vi "Project.vi"() -> ()   [LabVIEW 2023]
uses:
  WasherDryerControl.ctl
panel:
  out "Duration in hours":dbl
  out "Window":dbl(knob) scale=0.0..1000.0
  out "Temp":dbl
  out "Count":i32
  out "State":T1=enum."DO IT, ANAKIN"
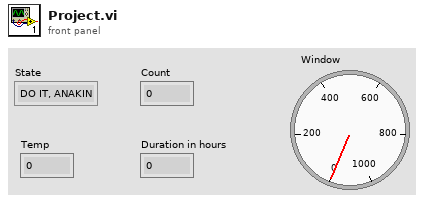
[diagram p1: front panel]
types:
  T1 = typedef "WasherDryerControl.ctl" = enum16{"Start", "Stop", "Wait", "Wash", "Cycle", "400", "800", "1200", "Temp", "Dry", "Heat", "Dry Flat", "Low heat", "High Heat", "Duration", "1h", "2h", "DO IT, ANAKIN"}
  T2 = enum16{"Left Button", "Center Button", "Right Button", "Window Close"}
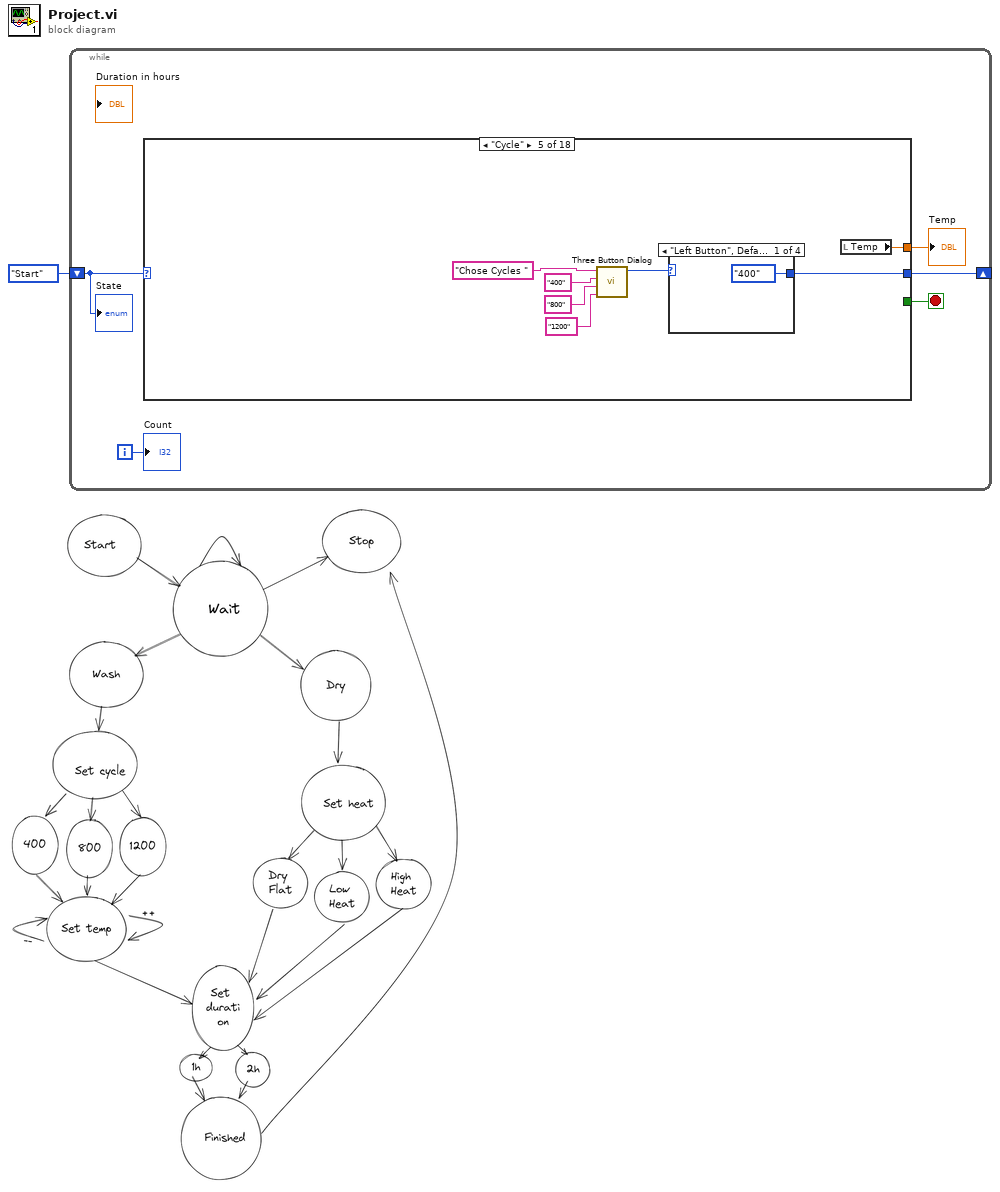
[diagram p0: block diagram]
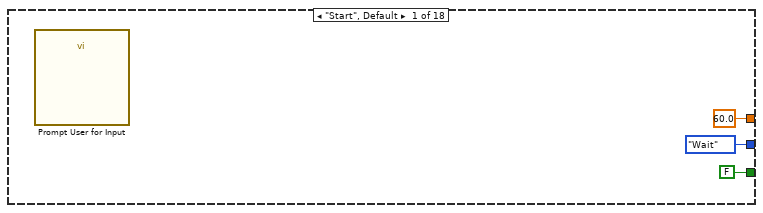
[diagram p2: hidden frame]
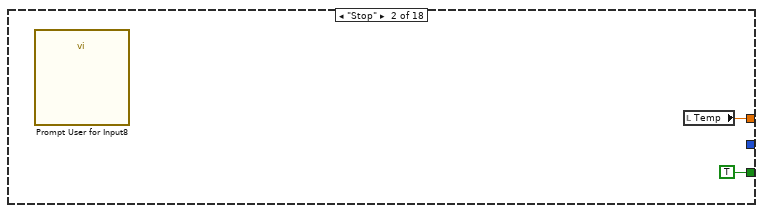
[diagram p3: hidden frame]
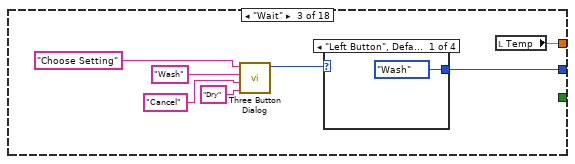
[diagram p4: hidden frame]
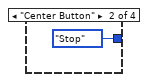
[diagram p5: hidden frame]
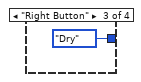
[diagram p6: hidden frame]
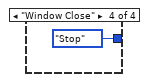
[diagram p7: hidden frame]
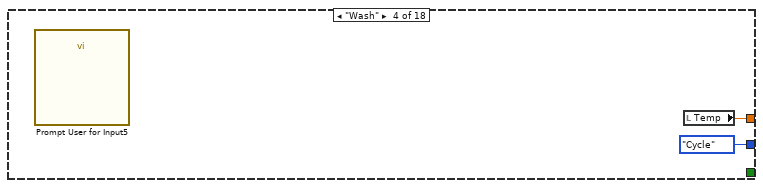
[diagram p8: hidden frame]
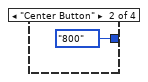
[diagram p9: hidden frame]
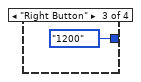
[diagram p10: hidden frame]
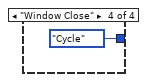
[diagram p11: hidden frame]
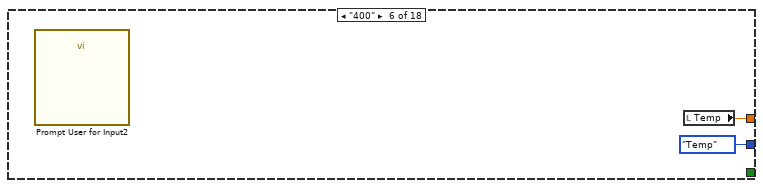
[diagram p12: hidden frame]
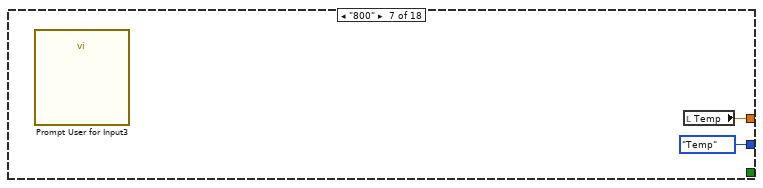
[diagram p13: hidden frame]
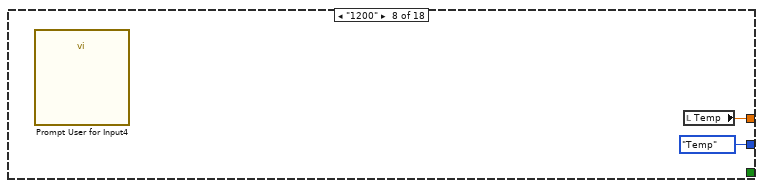
[diagram p14: hidden frame]
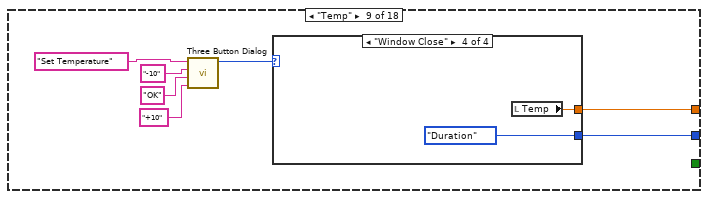
[diagram p15: hidden frame]
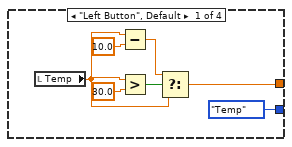
[diagram p16: hidden frame]
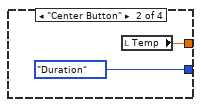
[diagram p17: hidden frame]
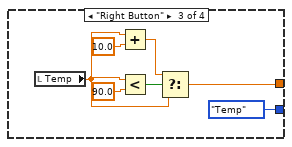
[diagram p18: hidden frame]
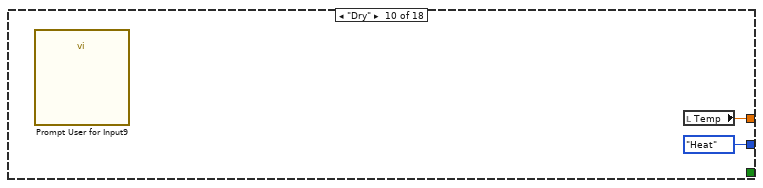
[diagram p19: hidden frame]
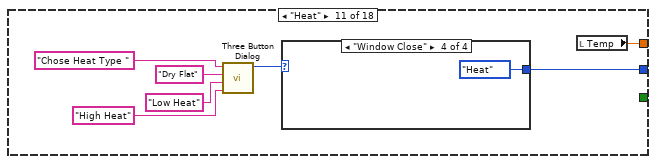
[diagram p20: hidden frame]
diagram:
  n1 = while {
    shift-right: [w3] -> _
    shift-left: WasherDryerControl."Start" ("Enum 2") -> [w4]
    i -> [w6]
    stop <- w5 stop-if-true
    n2 = case shown="\"Cycle\"" w4 {
      tunnel: [FALSE TRUE _ _ _ _ _ _ _ _ _ _ _ _ _ _ _ _] -> w5
      tunnel: [WasherDryerControl."Wait" ("Enum 2") _ w17 WasherDryerControl."Cycle" ("Enum 2") w29 WasherDryerControl."Temp" ("Enum 2") WasherDryerControl."Temp" ("Enum 2") WasherDryerControl."Temp" ("Enum 2") w43 WasherDryerControl."Heat" ("Enum 2") w70 WasherDryerControl."Duration" ("Enum 2") WasherDryerControl."Duration" ("Enum 2") WasherDryerControl."Duration" ("Enum 2") w87 WasherDryerControl."DO IT, ANAKIN" ("Enum 2") WasherDryerControl."DO IT, ANAKIN" ("Enum 2") w101] -> w3
      tunnel: [60.0 ("Temp") w10 w12 w23 w25 w36 w38 w40 w42 w67 w69 0.0 ("Temp") 30.0 ("Temp") 90.0 ("Temp") w86 w94 w97 w100] -> w2
      frame "Start", Default {
        n3 = call "Prompt User for Input"() -> ()  [unwired: 18 in, 2 out]
      }
      frame "Stop" {
        n4 = call "Prompt User for Input8"() -> ()  [unwired: 18 in, 2 out]
        n5 = local read "Temp"() -> (w10:dbl)
      }
      frame "Wait" {
        n6 = call <vilib>:"Three Button Dialog.vi"("Right Button Text (\"Cancel\")"="Dry" ("Right Button Text (\"Cancel\")"), "Center Button Text (\"No\")"="Cancel" ("Center Button Text (\"No\")"), "Left Button Text (\"Yes\")"="Wash" ("Left Button Text (\"Yes\")"), "message"="Choose Setting") -> ("Which Button?"=w18:T2)  [unwired: 7 in]
        n7 = case shown="\"Left Button\", Default" w18 {
          tunnel: [WasherDryerControl."Wash" ("Enum 2") WasherDryerControl."Stop" ("Enum 2") WasherDryerControl."Dry" ("Enum 2") WasherDryerControl."Stop" ("Enum 2")] -> w17
          frame "Left Button", Default {
          }
          frame "Center Button" {
          }
          frame "Right Button" {
          }
          frame "Window Close" {
          }
        }
        n8 = local read "Temp"() -> (w12:dbl)
      }
      frame "Wash" {
        n9 = call "Prompt User for Input5"() -> ()  [unwired: 18 in, 2 out]
        n10 = local read "Temp"() -> (w23:dbl)
      }
      frame "Cycle" {
        n11 = call <vilib>:"Three Button Dialog.vi"("Right Button Text (\"Cancel\")"="1200" ("Right Button Text (\"Cancel\")"), "Center Button Text (\"No\")"="800" ("Center Button Text (\"No\")"), "Left Button Text (\"Yes\")"="400" ("Center Button Text (\"No\")"), "message"="Chose Cycles ") -> ("Which Button?"=w31:T2)  [unwired: 7 in]
        n12 = case shown="\"Left Button\", Default" w31 {
          tunnel: [WasherDryerControl."400" ("Enum 2") WasherDryerControl."800" ("Enum 2") WasherDryerControl."1200" ("Enum 2") WasherDryerControl."Cycle" ("Enum 2")] -> w29
          frame "Left Button", Default {
          }
          frame "Center Button" {
          }
          frame "Right Button" {
          }
          frame "Window Close" {
          }
        }
        n13 = local read "Temp"() -> (w25:dbl)
      }
      frame "400" {
        n14 = call "Prompt User for Input2"() -> ()  [unwired: 18 in, 2 out]
        n15 = local read "Temp"() -> (w36:dbl)
      }
      frame "800" {
        n16 = call "Prompt User for Input3"() -> ()  [unwired: 18 in, 2 out]
        n17 = local read "Temp"() -> (w38:dbl)
      }
      frame "1200" {
        n18 = call "Prompt User for Input4"() -> ()  [unwired: 18 in, 2 out]
        n19 = local read "Temp"() -> (w40:dbl)
      }
      frame "Temp" {
        n20 = call <vilib>:"Three Button Dialog.vi"("Right Button Text (\"Cancel\")"="+10" ("Right Button Text (\"Cancel\")"), "Center Button Text (\"No\")"="OK" ("Center Button Text (\"No\")"), "Left Button Text (\"Yes\")"="-10" ("Left Button Text (\"Yes\")"), "message"="Set Temperature") -> ("Which Button?"=w44:T2)  [unwired: 7 in]
        n21 = case shown="\"Window Close\"" w44 {
          tunnel: [WasherDryerControl."Temp" ("Enum 2") WasherDryerControl."Duration" ("Enum 2") WasherDryerControl."Temp" ("Enum 2") WasherDryerControl."Duration" ("Enum 2")] -> w43
          tunnel: [w50 w56 w59 w65] -> w42
          frame "Left Button", Default {
            n22 = local read "Temp"() -> (w51:dbl)
            n23 = Subtract(x=w51, y=10.0) -> (x-y=w53:dbl)
            n24 = Greater?(x=w51, y=30.0) -> (0:w54:bool)
            n25 = Select(t=w53, s=w54, f=w51) -> (s? t:f=w50:dbl)
          }
          frame "Center Button" {
            n26 = local read "Temp"() -> (w56:dbl)
          }
          frame "Right Button" {
            n27 = local read "Temp"() -> (w60:dbl)
            n28 = Add(x=w60, y=10.0) -> (x+y=w62:dbl)
            n29 = Less?(x=w60, y=90.0) -> (x < y?=w63:bool)
            n30 = Select(t=w62, s=w63, f=w60) -> (s? t:f=w59:dbl)
          }
          frame "Window Close" {
            n31 = local read "Temp"() -> (w65:dbl)
          }
        }
      }
      frame "Dry" {
        n32 = call "Prompt User for Input9"() -> ()  [unwired: 18 in, 2 out]
        n33 = local read "Temp"() -> (w67:dbl)
      }
      frame "Heat" {
        n34 = call <vilib>:"Three Button Dialog.vi"("Right Button Text (\"Cancel\")"="High Heat" ("Right Button Text (\"Cancel\")"), "Center Button Text (\"No\")"="Low Heat" ("Center Button Text (\"No\")"), "Left Button Text (\"Yes\")"="Dry Flat" ("Center Button Text (\"No\")"), "message"="Chose Heat Type ") -> ("Which Button?"=w75:T2)  [unwired: 7 in]
        n35 = case shown="\"Window Close\"" w75 {
          tunnel: [WasherDryerControl."Dry Flat" ("Enum 2") WasherDryerControl."Low heat" ("Enum 2") WasherDryerControl."High Heat" ("Enum 2") WasherDryerControl."Heat" ("Enum 2")] -> w70
          frame "Left Button", Default {
          }
          frame "Center Button" {
          }
          frame "Right Button" {
          }
          frame "Window Close" {
          }
        }
        n36 = local read "Temp"() -> (w69:dbl)
      }
      frame "Dry Flat" {
        n37 = call "Prompt User for Input10"() -> ()  [unwired: 18 in, 2 out]
      }
      frame "Low heat" {
        n38 = call "Prompt User for Input11"() -> ()  [unwired: 18 in, 2 out]
      }
      frame "High Heat" {
        n39 = call "Prompt User for Input12"() -> ()  [unwired: 18 in, 2 out]
      }
      frame "Duration" {
        n40 = Two Button Dialog(message="Choose Duration", 1:"Long (2 hours)" ("F button name (\"Cancel\")"), 2:"Short (1 hour)" ("T button name (\"OK\")")) -> (T button?=w90:bool)
        n41 = Select(t=WasherDryerControl."1h" ("Enum 2"), s=w90, f=WasherDryerControl."2h" ("Enum 2")) -> (s? t:f=w87:T1)
        n42 = local read "Temp"() -> (w86:dbl)
      }
      frame "1h" {
        n43 = call "Prompt User for Input6"() -> ()  [unwired: 18 in, 2 out]
        n44 = local write "Duration in hours"(1.0 ("Duration in hours")) -> ()
        n45 = local read "Temp"() -> (w94:dbl)
      }
      frame "2h" {
        n46 = call "Prompt User for Input7"() -> ()  [unwired: 18 in, 2 out]
        n47 = local write "Duration in hours"(2.0 ("Duration in hours")) -> ()
        n48 = local read "Temp"() -> (w97:dbl)
      }
      frame "DO IT, ANAKIN" {
        n49 = flat-sequence {
          tunnel: [WasherDryerControl."Stop" ("Enum 2")] -> w101
          frame #0 {
            n50 = for {
              N: 1000 -> [_]
              i -> [w106]
              n51 = local read "Duration in hours"() -> (w105:dbl)
              n52 = Multiply(x=u32 10 ("milliseconds to wait"), y=w105) -> (x*y=w103:dbl)
              n53 = Wait (ms)(milliseconds to wait=w103) -> ()  [unwired: 1 out]
              "Window" <- w106
            }
          }
          frame #1 {
          }
        }
        n54 = local read "Temp"() -> (w100:dbl)
      }
    }
    "Temp" <- w2
    "State" <- w4
    "Count" <- w6
  }
